vi "Reformat Message.vi"(8 "error in (no error)":errorcluster, 11 "TCS in":refnum<class "TCS.lvclass">) -> (0 "error out":errorcluster, 3 "TCS out":refnum<class "TCS.lvclass">)   [LabVIEW 2018, in "TCS.lvclass"]
uses:
  TCS.lvclass
  <vilib>/Utility/error.llb/whitespace.ctl
  TCS.lvclass/TCS.ctl
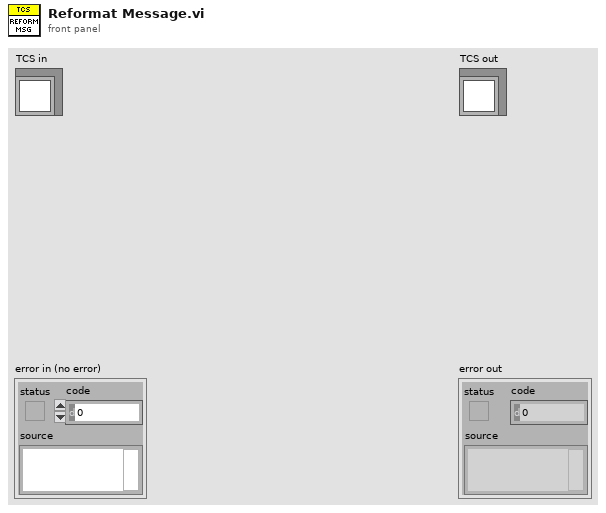
[diagram p1: front panel]
types:
  T1 = typedef "whitespace.ctl" = u16
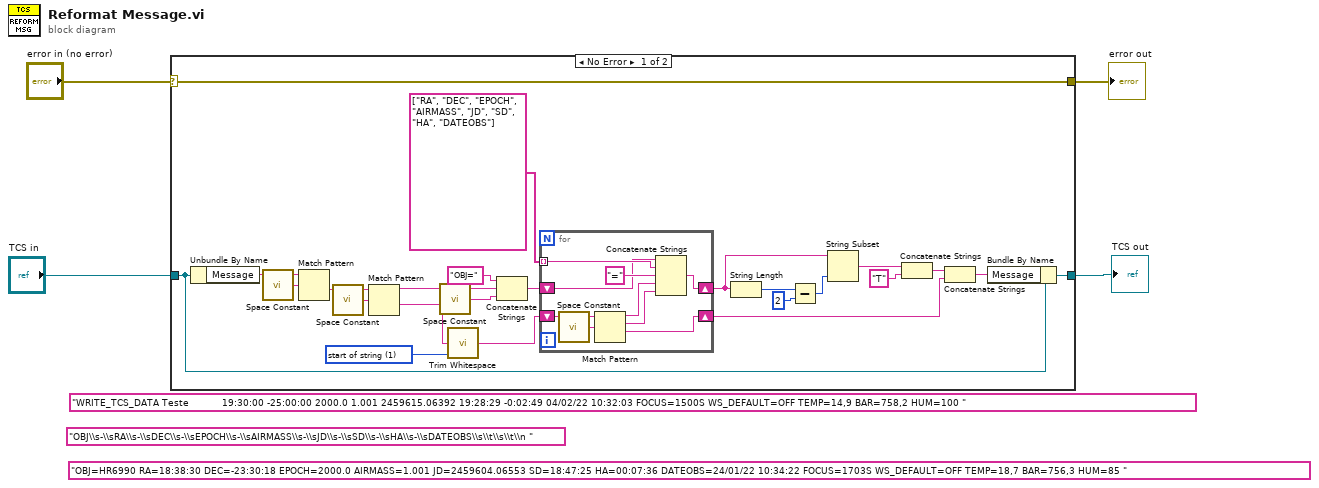
[diagram p0: block diagram]
diagram:
  (unwired) "OBJ=HR6990 RA=18:38:30 DEC=-23:30:18 EPOCH=2000.0 AIRMASS=1.001 JD=2459604.06553 SD=18:47:25 HA=00:07:36 DATEOBS=24/01/22 10:34:22 FOCUS=1703S WS_DEFAULT=OFF TEMP=18,7 BAR=756,3 HUM=85 "
  (unwired) "OBJ\\s-\\sRA\\s-\\sDEC\\s-\\sEPOCH\\s-\\sAIRMASS\\s-\\sJD\\s-\\sSD\\s-\\sHA\\s-\\sDATEOBS\\s\\t\\s\\t\\n "
  (unwired) "WRITE_TCS_DATA Teste           19:30:00 -25:00:00 2000.0 1.001 2459615.06392 19:28:29 -0:02:49 04/02/22 10:32:03 FOCUS=1500S WS_DEFAULT=OFF TEMP=14,9 BAR=758,2 HUM=100 "
  n1 = case shown="No Error" "error in (no error)" {
    selector: "error in (no error)" -> [w28 w39]
    tunnel: [w28 w39] -> w3
    tunnel: [w22 w38] -> w1
    tunnel: "TCS in" -> [w23 w38]
    frame No Error {
      w8 = T1 1 items=["both", "start of string", "end of string"] ("location (both)")
      n2 = Unbundle By Name(w23) -> ("Message"=w5:string)
      n3 = call <vilib>:"Space Constant.vi"() -> ("String"=w20:string)
      n4 = Match Pattern(string=w5, regular expression=w20) -> (after substring=w19:string)  [unwired: 1 in, 3 out]
      n5 = call <vilib>:"Space Constant.vi"() -> ("String"=w10:string)
      n6 = Match Pattern(string=w19, regular expression=w10) -> (before substring=w9:string, after substring=w7:string)  [unwired: 1 in, 2 out]
      n7 = call <vilib>:"Space Constant.vi"() -> ("String"=w26:string)
      n8 = call <vilib>:"Trim Whitespace.vi"("string"=w7, "location (both)"=w8) -> ("trimmed string"=w6:string)
      n9 = Concatenate Strings("OBJ=", w9, w26) -> (w24:string)
      n10 = for {
        tunnel: string[] ["RA", "DEC", "EPOCH", "AIRMASS", "JD", "SD", "HA", "DATEOBS"] -> [w33] mode=indexing
        shift-right: [w32] -> w11
        shift-left: w24 -> [w29]
        shift-right: [w31] -> w12
        shift-left: w6 -> [w37]
        n11 = call <vilib>:"Space Constant.vi"() -> ("String"=w36:string)
        n12 = Match Pattern(string=w37, regular expression=w36) -> (before substring=w35:string, match substring=w30:string, after substring=w31:string)  [unwired: 1 in, 1 out]
        n13 = Concatenate Strings(w29, w33, "=", w35, w30) -> (w32:string)
      }
      n14 = String Length(string=w11) -> (length=w18:i32)
      n15 = Subtract(x=w18, y=2) -> (x-y=w16:i32)
      n16 = String Subset(string=w11, length (rest)=w16) -> (substring=w15:string)  [unwired: 1 in]
      n17 = Concatenate Strings(w15, "T") -> (w13:string)
      n18 = Concatenate Strings(w13, w12) -> (w21:string)
      n19 = Bundle By Name(cluster=w23, "Message"=w21) -> (w22:refnum<class "TCS.lvclass">)
    }
    frame Error {
    }
  }
  "error out" <- w3
  "TCS out" <- w1
